vi "Default Splitter Positions.vi"() -> (2 "Splitter Positions":i32[](array[numeric]))   [LabVIEW 2023, in "Manual UI.lvlib" / "Manual UI.lvclass"]
uses:
  Project/Manual UI.lvclass
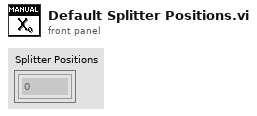
[diagram p1: front panel]
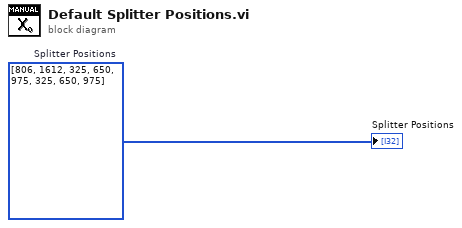
[diagram p0: block diagram]
diagram:
  w1 = i32[] [806, 1612, 325, 650, 975, 325, 650, 975]  # Splitter Positions
  "Splitter Positions" <- w1
